vi "Write.vi"(8 "error in (no error)":errorcluster, 10 "Log Data":T1={"Time"=timestamp(0 s since 1904-01-01), "Level"=enum."INFO", "Logger"="", "Message"="", "Arguments"=[]} {"Time" format="%<%x %.3X>T"}, 11 "SQLite Database in":refnum<class "SQLite Database.lvclass">) -> (0 "error out":errorcluster, 3 "SQLite Database out":refnum<class "SQLite Database.lvclass">)   [LabVIEW 2019, in "TSC Event Logger.lvlib" / "SQLite Database.lvclass"]
uses:
  SQLite Database.lvclass
  C:/Development/Reuse-libraries/Event Logger/Log Sinks/Log Sinks.lvclass
  Log Data.ctl
  Log/Event Level.ctl
  SQLite Database.lvclass/SQLite Database.ctl
  <vilib>/drjdpowell/SQLite Library/SQL Statement/SQL Statement.lvclass/SQL Statement.ctl
  <vilib>/drjdpowell/SQLite Library/SQL Statement/Bind Text.vi
  <vilib>/drjdpowell/SQLite Library/SQL Statement/Step.vi
  <vilib>/drjdpowell/SQLite Library/SQL Statement/Error Message.vi
  <vilib>/drjdpowell/SQLite Library/SQL Statement/SQL Statement.lvclass
  Log Sinks.lvclass
  TSC Event Logger.lvlib
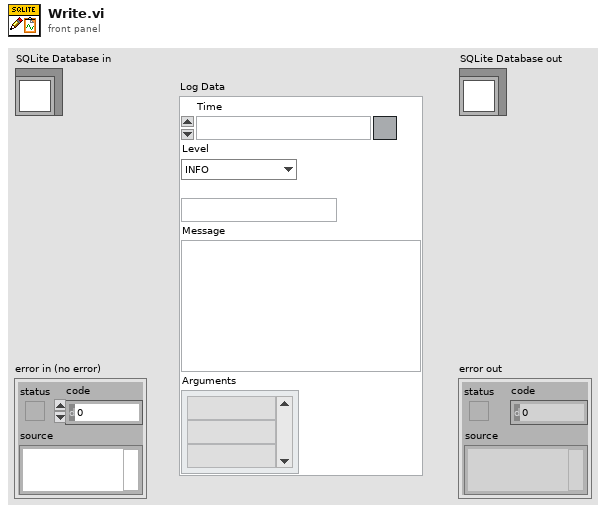
[diagram p1: front panel]
types:
  T1 = typedef "TSC Event Logger.lvlib/Log Data.ctl" = cluster{"Time":timestamp, "Level":T2, "Logger":string, "Message":string, "Arguments":string[]}
  T2 = typedef "TSC Event Logger.lvlib/Event Level.ctl" = enum16{"OFF", "TRACE", "DEBUG", "INFO", "WARN", "ERROR", "FATAL"}
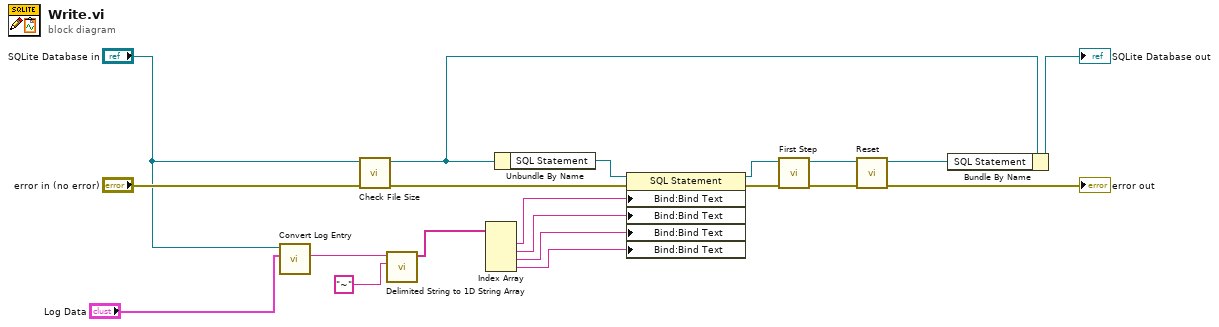
[diagram p0: block diagram]
diagram:
  n1 = call "Convert Log Entry.vi"("Log Data"="Log Data", "Log Sink in"="SQLite Database in") -> ("Log Entry"=w10:string)  [unwired: 9 in]
  n2 = call "Check File Size.vi"("error in (no error)"="error in (no error)", "SQLite Database in"="SQLite Database in") -> ("error out"=w3:errorcluster, "SQLite Database out"=w1:refnum<class "SQLite Database.lvclass">)  [unwired: 8 in]
  n3 = call <vilib>:"Delimited String to 1D String Array.vi"("delimiter"="~", "delimited string"=w10) -> ("string array"=w8:string[])  [unwired: 9 in]
  n4 = Index Array(array=w8) -> (element #1=w7:string, element #2=w6:string, element #3=w5:string, element #4=w4:string)  [unwired: 4 in]
  n5 = Unbundle By Name(w1) -> ("SQL Statement"=w18:refnum<class "SQL Statement.lvclass">)
  n6 = property class="SQL Statement"(reference=w18, error in=w3, "Bind:Bind Text"=w7, "Bind:Bind Text"=w6, "Bind:Bind Text"=w5, "Bind:Bind Text"=w4) -> (reference out=w14:refnum<class "SQL Statement.lvclass">, error out=w19:errorcluster)
  n7 = call <vilib>:"First Step.vi"("error in (no error)"=w19, "SQL Statement in"=w14) -> ("error out"=w17:errorcluster, "SQL Statement"=w15:refnum<class "SQL Statement.lvclass">)  [unwired: 7 in, 1 out]
  n8 = call <vilib>:"Reset.vi"("error in (no error)"=w17, "SQL Statement in"=w15) -> ("error out"=→"error out":errorcluster, "SQL Statement"=w12:refnum<class "SQL Statement.lvclass">)  [unwired: 8 in]
  n9 = Bundle By Name(cluster=w1, "SQL Statement"=w12) -> (→"SQLite Database out":refnum<class "SQLite Database.lvclass">)
